vi "Load DLL.vi"(8 "error in (no error)":errorcluster, 9 "BL Finder DLL Path":path, 10 "DLL Path":path, 11 "Potentiostat Galvanostat in":refnum<class "Potentiostat Galvanostat.lvclass">) -> (0 "error out":errorcluster, 3 "Potentiostat Galvanostat out":refnum<class "Potentiostat Galvanostat.lvclass">)   [LabVIEW 2018, in "Potentiostat Galvanostat.lvclass"]
uses:
  Potentiostat Galvanostat.lvclass
  Controls/Error Codes.ctl
  Potentiostat Galvanostat.lvclass/Potentiostat Galvanostat.ctl
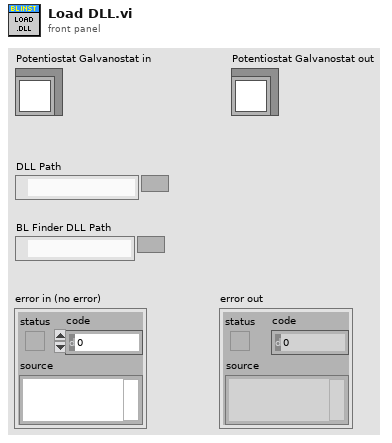
[diagram p1: front panel]
types:
  T1 = typedef "Potentiostat Galvanostat.lvclass/Error Codes.ctl" = i32
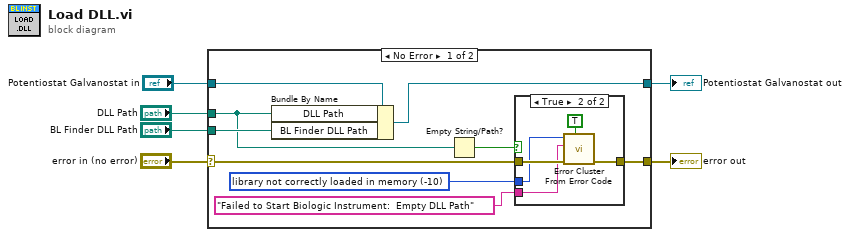
[diagram p0: block diagram]
diagram:
  n1 = case shown="No Error" "error in (no error)" {
    selector: "error in (no error)" -> [w12 w23]
    tunnel: [w11 w23] -> w5
    tunnel: [w14 w22] -> w3
    tunnel: "Potentiostat Galvanostat in" -> [w15 w22]
    tunnel: "DLL Path" -> [w10 _]
    tunnel: "BL Finder DLL Path" -> [w13 _]
    frame No Error {
      w8 = T1 -10 items=["No error found"=0, "invalid function parameters"=-4, "library not correctly loaded in memory"=-10] ("Error Code")
      n2 = Bundle By Name(cluster=w15, "DLL Path"=w10, "BL Finder DLL Path"=w13) -> (w14:refnum<class "Potentiostat Galvanostat.lvclass">)
      n3 = Empty String/Path?(string/path=w10) -> (empty?=w9:bool)
      n4 = case shown="True" w9 {
        tunnel: w12 -> [w16 w21]
        tunnel: [w16 w19] -> w11
        tunnel: w8 -> [_ w18]
        tunnel: "Failed to Start Biologic Instrument:  Empty DLL Path" -> [_ w17]
        frame False {
        }
        frame True {
          n5 = call <vilib>:"Error Cluster From Error Code.vi"("show call chain? (False)"=TRUE, "error in (no error)"=w21, "error message (\"\")"=w17, "error code (0)"=w18) -> ("error out"=w19:errorcluster)  [unwired: 5 in]
        }
      }
    }
    frame Error {
    }
  }
  "error out" <- w5
  "Potentiostat Galvanostat out" <- w3
